vi "Configure Output Protection.vi"(7 "Over Current Protection Delay (0.02 seconds)":dbl=0.02 format="%^.3g", 8 "error in (no error)":errorcluster {"code" format="%.0x"}, 9 "Enable Coupling (False)":bool, 10 "Channel Name (1)":string="1", 11 "VISA resource name":refnum<visa-resource-name>) -> (0 "error out":errorcluster {"code" format="%.0x"}, 3 "VISA resource name out":refnum<visa-resource-name>)   [LabVIEW 2014, in "Agilent N6700 Series.lvlib"]
doc: "Sets the coupling status and over current protection (OCP) delay."
uses:
  Agilent N6700 Series.lvlib
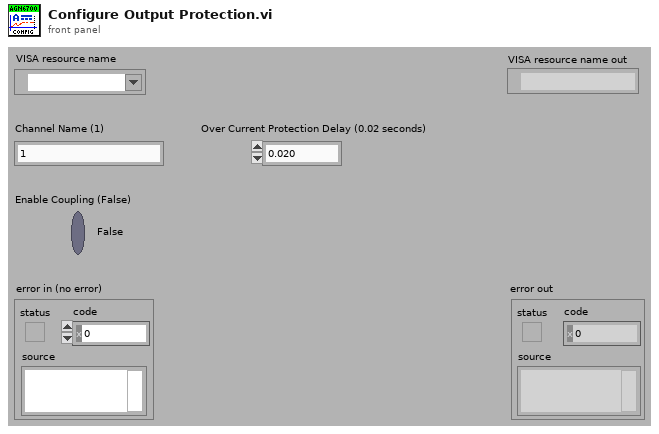
[diagram p1: front panel]
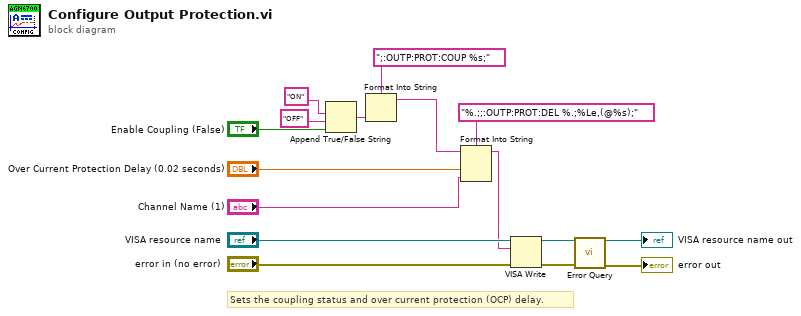
[diagram p0: block diagram]
diagram:
  # "Sets the coupling status and over current protection (OCP) delay."
  n1 = Append True/False String(1:"Enable Coupling (False)", 2:"OFF", 3:"ON") -> (0:w8:string)  [unwired: 1 in]
  n2 = Format Into String(format string=";:OUTP:PROT:COUP %s;", w8) -> (resulting string=w4:string)  [unwired: 2 in, 1 out]
  n3 = Format Into String(format string="%.;;:OUTP:PROT:DEL %.;%Le,(@%s);", initial string=w4, "Over Current Protection Delay (0.02 seconds)", "Channel Name (1)") -> (resulting string=w2:string)  [unwired: 1 in, 1 out]
  n4 = VISA Write(VISA resource name="VISA resource name", write buffer=w2, error in (no error)="error in (no error)") -> (VISA resource name out=w12:refnum<visa-resource-name>, error out=w11:errorcluster)  [unwired: 1 out]
  n5 = call "Error Query.vi"("VISA resource name"=w12, "error in (no error)"=w11) -> ("VISA resource name out"=→"VISA resource name out":refnum<visa-resource-name>, "error out"=→"error out":errorcluster)  [unwired: 10 in, 2 out]
